vi "_Import Data.vi"(4 "error in (no error)":errorcluster, 7 "file path (dialog if empty)":path) -> (0 "error out":errorcluster, 1 "Spectrum":i32[](array[numeric]), 2 "Masses":dbl[](array[numeric]), 3 "2D data":dbl[][](array[numeric]) format="%0.2f")   [LabVIEW 2015]
doc: "Converts a 2D or 1D array of single-precision numbers to a text string and writes the string to a new byte stream file or appends the string to an existing file."
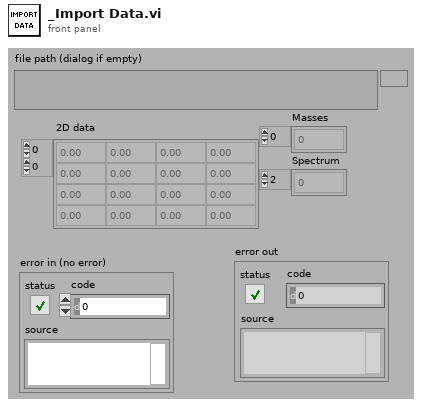
[diagram p1: front panel]
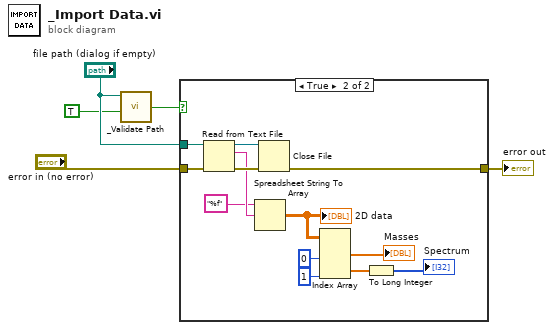
[diagram p0: block diagram]
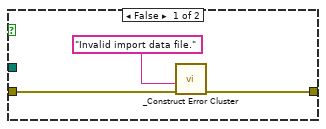
[diagram p2: hidden frame]
diagram:
  n1 = call "_Validate Path.vi"("Check Exist (F)"=TRUE, "path"="file path (dialog if empty)") -> ("Valid"=w1:bool)  [unwired: 2 in]
  n2 = case shown="True" w1 {
    tunnel: "error in (no error)" -> [w7 w17]
    tunnel: [w6 w16] -> w4
    tunnel: "file path (dialog if empty)" -> [_ w9]
    frame False {
      n3 = call "_Construct Error Cluster.vi"("error in"=w7, "reason"="Invalid import data file.") -> ("error out"=w6:errorcluster)  [unwired: 2 in, 3 out]
    }
    frame True {
      n4 = Read from Text File(file (use dialog)=w9, error in=w17) -> (refnum out=w20:refnum<file>, text=w19:string, error out=w21:errorcluster)  [unwired: 2 in, 1 out]
      n5 = Spreadsheet String To Array(format string="%f" ("format (%.3f)"), spreadsheet string=w19) -> (array=w15:dbl[][])  [unwired: 2 in]
      "2D data" <- w15
      n6 = Close File(refnum=w20, error in=w21) -> (error out=w16:errorcluster)  [unwired: 1 out]
      n7 = Index Array(array=w15, index (col) #1=0 ("disabled index (col)"), index (col) #2=1 ("index (col)")) -> (element #1=→"Masses":dbl[], element #2=w11:dbl[])  [unwired: 2 in]
      n8 = To Long Integer(number=w11) -> (32bit integer=→"Spectrum":i32[])
    }
  }
  "error out" <- w4
